vi "VideoRecording.vi"() -> ()   [LabVIEW 2015]
doc: "The LL Ring VI acquires images continuously and displays them in an image control using the low-level acquisition VIs. A ring initiates a continuous high-speed acquisition to multiple buffers and is appropriate for high-speed applications that perform processing on every image. Multiple buffers are useful when processing times vary depending on other applications and processing results .\n\nIMAQ Init initializes the device. IMAQ Configure List configures the buffer list with multiple buffers. IMAQ Create creates the image buffers. Call IMAQ Configure Buffer once for each buffer in the buffer list. IMAQ Start starts the acquisition, and IMAQ Extract Buffer ensures that the current image is not overwritten. An image control displays the image on the front panel. After exiting the loop, IMAQ Extract Buffer releases the last extracted buffer. IMAQ Close releases resources associated with the acquisition, and IMAQ Dispose frees the image buffer."
uses:
  <vilib>/vision/Avi.llb/IMAQ AVI2 Refnum.ctl
  <vilib>/vision/Avi.llb/IMAQ AVI2 Codec Path.ctl
  SubVI/Global_Video_Frame_Number.vi
panel:
  in  "Frames per file":i32=6000
  out "AVI Refnum":T1
  out "Video recording":bool=TRUE
  in  "Record? (Home bt.)":bool
  in  "codec index":i32=5
  out "Error (%)":dbl format="%#.4g"
  out "Missing Frames":i32
  out "Frame Number":u32=4950121
  out "codec":string="Y800 Uncompressed Grey Scale (NI Vision)"
  in  "AVI File Path":path=path "E:/Video/4/200fps.avi"
  out "Processed Frames/s":dbl=200.0 format="%#.1g"
  in  "Stop":bool
  out "Saved Frames":i32=21551
  out "Image":T2(plugin-control)
  in  "camera selection":string="img0"
  in  "Buffer size (frames)":u32=1000
  # "ToDo:\n - add JSON output\n - andd indicator of _s# number"
  # "1.  Initialisation"
  # "Codec should be:\n\"Y800 Uncompressed Grey Scale\""
  # "Naming convention:\n - use the name above and add _s#.avi for videos\n - specs for saved videos is specified in name.json"
  # "2.  Recording"
  # "y"
  # "Record"
  # "x"
  # "Just Observe"
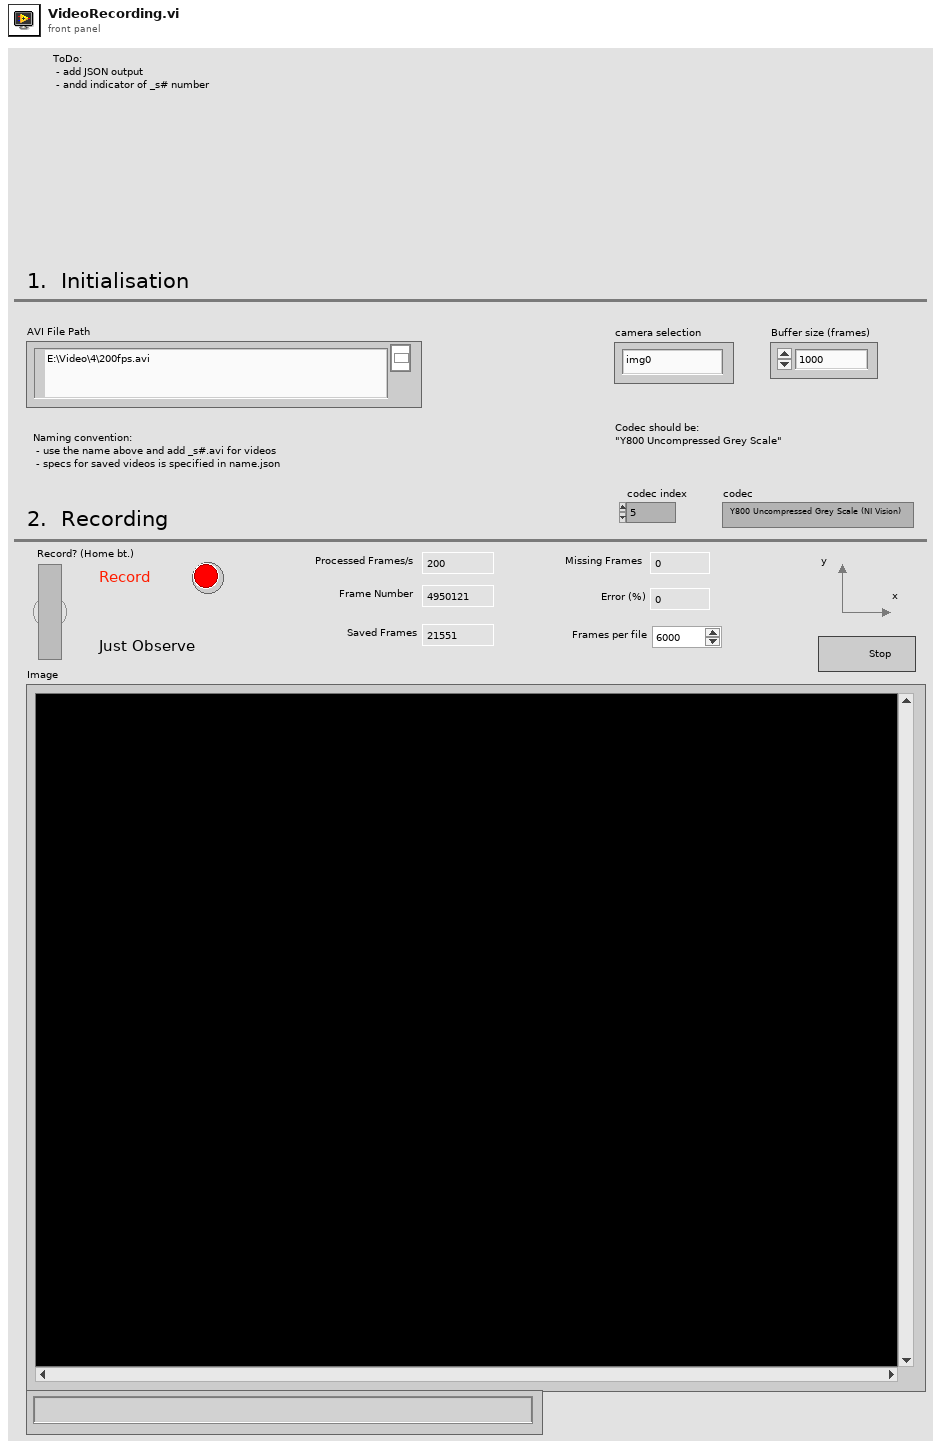
[diagram p1: front panel]
types:
  T1 = typedef "IMAQ AVI2 Refnum.ctl" = refnum<k20>
  T2 = typedef "IMAQ Image.ctl" = refnum<image>
  T3 = typedef "IMAQ AVI2 Codec Path.ctl" = u32
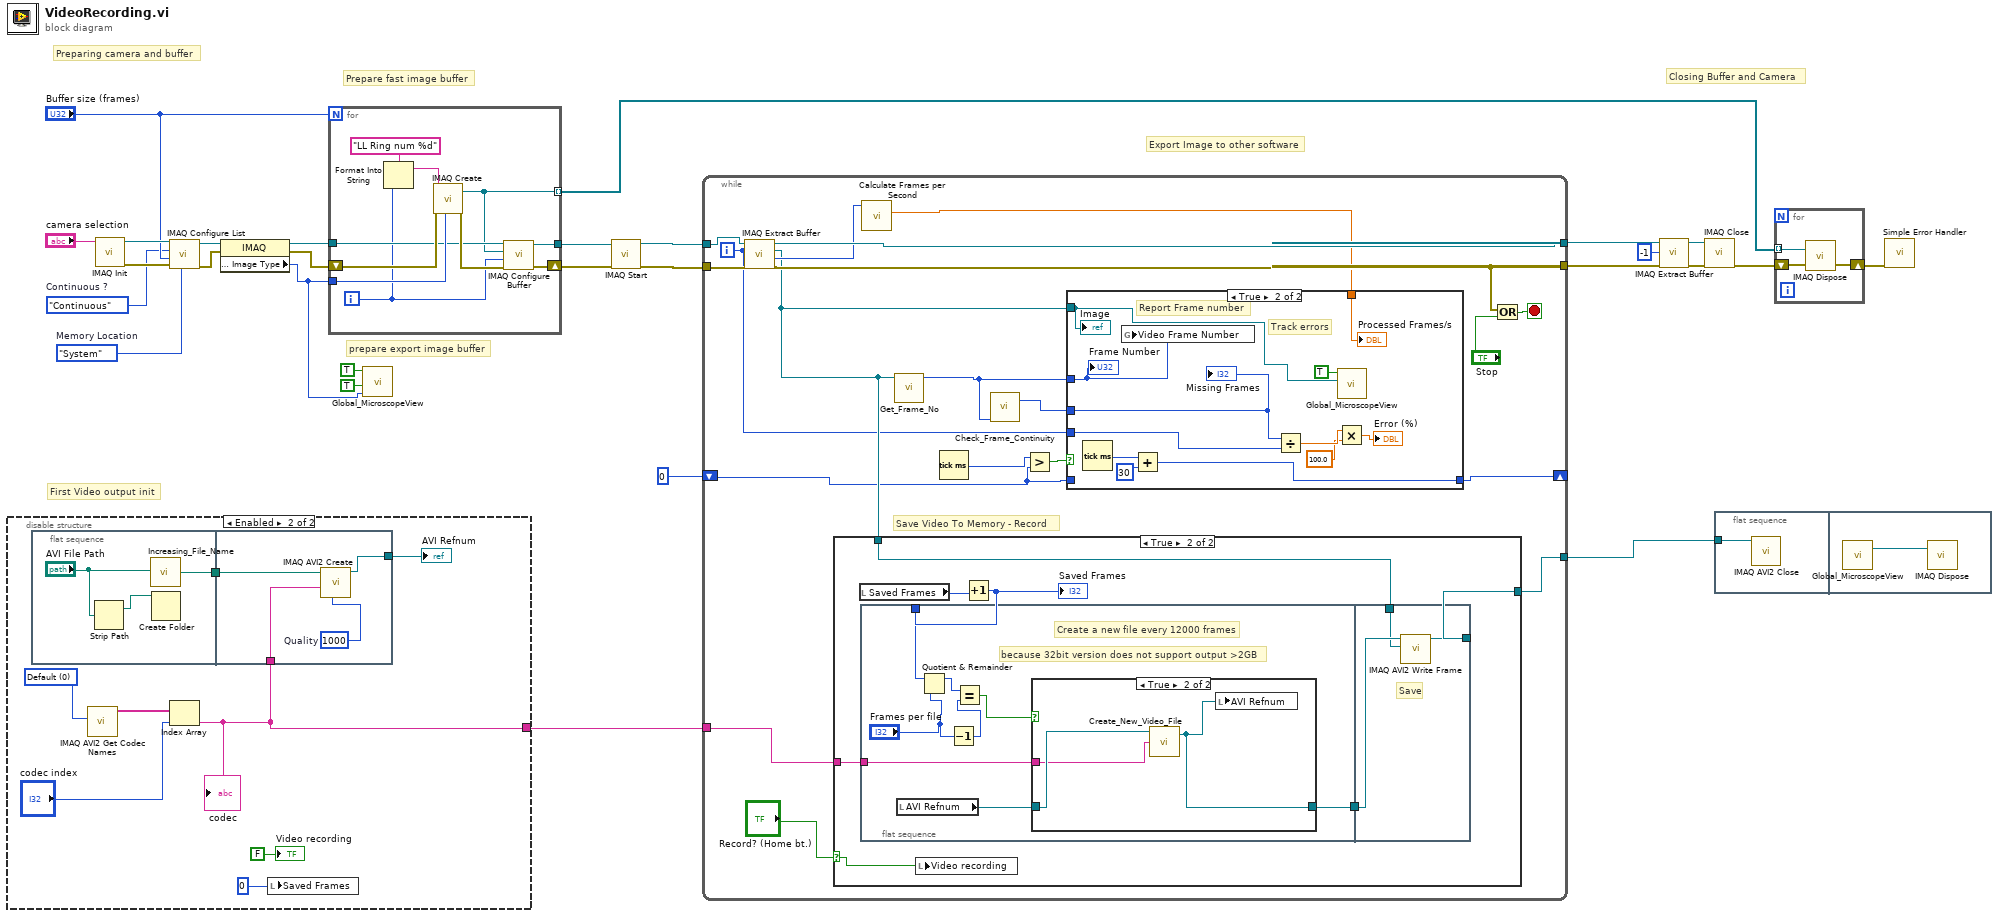
[diagram p0: block diagram]
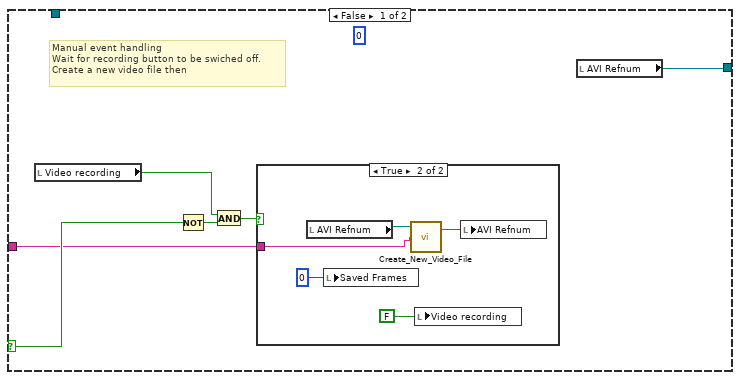
[diagram p4: hidden frame]
diagram:
  w10 = enum16{"System", "Onboard"}."System"  # Memory Location
  w9 = enum16{"One-Shot", "Continuous"}."Continuous"  # Continuous ?
  # "Export Image to other software"
  # "prepare export image buffer"
  # "Prepare fast image buffer"
  # "First Video output init"
  # "Closing Buffer and Camera"
  # "Preparing camera and buffer"
  n1 = disable-structure shown="Enabled" {
    disable-tunnel: [_ w29] -> w5
    frame Disabled {
    }
    frame Enabled {
      w36 = T3 0 items=["Default", "System", "Built in Vision"] ("Codec Source")
      n2 = flat-sequence {
        tunnel: [w39] -> w31
        tunnel: w31 -> [w41]
        tunnel: [w42] -> w30
        tunnel: w29 -> [w40]
        frame #0 {
          n3 = Strip Path(path="AVI File Path") -> (stripped path=w38:path)  [unwired: 1 out]
          n4 = call "Increasing_File_Name.vi"("Base AVI  path"="AVI File Path") -> ("Final AVI path"=w39:path)
          n5 = Create Folder(path (use dialog)=w38) -> ()  [unwired: 2 in, 3 out]
        }
        frame #1 {
          w43 = 1000  # Quality
          n6 = call "IMAQ AVI2 Create"("Quality"=w43, "Codec"=w40, "AVI Path"=w41) -> ("AVI Refnum"=w42:T1)  [unwired: 7 in, 1 out]
        }
      }
      n7 = call "IMAQ AVI2 Get Codec Names"("Codec Source"=w36) -> ("Codec Names"=w35:string[])  [unwired: 9 in, 1 out]
      n8 = Index Array(array=w35, index="codec index") -> (element=w29:string)
      "codec" <- w29
      n9 = local write "Saved Frames"(0 ("Saved Frames")) -> ()
      "AVI Refnum" <- w30
      "Video recording" <- FALSE ("Video recording")
    }
  }
  n10 = call <vilib>:"IMAQ Init.vi"("Interface Name"="camera selection") -> ("error out"=w27:errorcluster, "IMAQ Session Out"=w28:refnum<k11>)  [unwired: 1 in, 8 out]
  n11 = call <vilib>:"IMAQ Configure List.vi"("Memory Location"=w10, "error in (no error)"=w27, "Number of buffers"="Buffer size (frames)", "Continuous?"=w9, "IMAQ Session In"=w28) -> ("error out"=w23:errorcluster, "IMAQ Session Out"=w22:refnum<k11>)  [unwired: 1 in, 4 out]
  n12 = property class="IMAQ"(reference=w22, error in=w23) -> (reference out=w15:refnum<k11>, error out=w14:errorcluster, "Image Parameters : Image Type"=w2:u32)
  n13 = for {
    N: "Buffer size (frames)" -> [_]
    tunnel: [w53] -> w12
    tunnel: w2 -> [w51]
    tunnel: w15 -> [w48]
    shift-right: [w52] -> w11
    shift-left: w14 -> [w50]
    tunnel: [w44] -> w8 mode=indexing
    i -> [w45]
    n14 = Format Into String(format string="LL Ring num %d", w45) -> (resulting string=w47:string)  [unwired: 2 in, 1 out]
    n15 = call "IMAQ Create"("Image Name"=w47, "Image Type"=w51, "error in (no error)"=w50) -> ("New Image"=w44:T2, "error out"=w49:errorcluster)  [unwired: 1 in, 1 out]
    n16 = call <vilib>:"IMAQ Configure Buffer.vi"("error in (no error)"=w49, "Buffer Number"=w45, "Image In"=w44, "IMAQ Session In"=w48) -> ("error out"=w52:errorcluster, "IMAQ Session Out"=w53:refnum<k11>)  [unwired: 2 in, 4 out]
  }
  n17 = call "Global_MicroscopeView.vi"("Image Type"=w2, "Initialise"=TRUE, "Update Image"=TRUE) -> ()  [unwired: 1 in, 2 out]
  n18 = call <vilib>:"IMAQ Start.vi"("error in (no error)"=w11, "IMAQ Session In"=w12) -> ("error out"=w7:errorcluster, "IMAQ Session Out"=w18:refnum<k11>)  [unwired: 8 out]
  n19 = while {
    tunnel: [w70] -> w20
    tunnel: w18 -> [w71]
    tunnel: [w64] -> w19
    tunnel: w7 -> [w67]
    tunnel: [w63] -> w6
    tunnel: w5 -> [w62]
    shift-right: [w54] -> _
    shift-left: 0 -> [w55]
    i -> [w59]
    stop <- w72 stop-if-true
    # "Save Video To Memory - Record"
    n20 = call <vilib>:"IMAQ Extract Buffer.vi"("error in (no error)"=w67, "Buffer to extract"=w59, "IMAQ Session In"=w71) -> ("error out"=w64:errorcluster, "Buffer Number"=w68:i32, "Image Out"=w60:T2, "IMAQ Session Out"=w70:refnum<k11>)  [unwired: 5 out]
    n21 = case shown="True" "Record? (Home bt.)" {
      selector: "Record? (Home bt.)" -> [w88 w99]
      tunnel: [w91 w102] -> w63
      tunnel: w60 -> [_ w100]
      tunnel: w62 -> [w86 w98]
      frame False {
        (unwired) 0
        # "Manual event handling\nWait for recording button to be swiched off.\nCreate a new video file then"
        n22 = local read "Video recording"() -> (w87:bool)
        n23 = Not(x=w88) -> (.not. x?=w89:bool)
        n24 = And(x=w87, y=w89) -> (x .and. y?=w90:bool)
        n25 = case shown="True" w90 {
          tunnel: w86 -> [_ w92]
          frame False {
          }
          frame True {
            n26 = local read "AVI Refnum"() -> (w95:T1)
            n27 = local write "Saved Frames"(0 ("Saved Frames")) -> ()
            n28 = call "Create_New_Video_File.vi"("Codec"=w92, "AVI Refnum IN"=w95) -> ("AVI Refnum OUT"=w96:T1)  [unwired: 1 in, 1 out]
            n29 = local write "Video recording"(FALSE ("Video recording")) -> ()
            n30 = local write "AVI Refnum"(w96) -> ()
          }
        }
        n31 = local read "AVI Refnum"() -> (w91:T1)
      }
      frame True {
        n32 = local read "Saved Frames"() -> (w103:i32)
        n33 = flat-sequence {
          tunnel: w97 -> [w109]
          tunnel: [w106] -> w101
          tunnel: w98 -> [w105]
          tunnel: [w118] -> w102
          tunnel: w101 -> [w117]
          tunnel: w100 -> [w116]
          frame #0 {
            # "because 32bit version does not support output >2GB"
            # "Create a new file every 12000 frames"
            n34 = local read "AVI Refnum"() -> (w107:T1)
            n35 = Quotient & Remainder(x=w109, y="Frames per file") -> (x-y*floor(x/y)=w111:i32)  [unwired: 1 out]
            n36 = Decrement(x="Frames per file") -> (x-1=w110:i32)
            n37 = Equal?(x=w111, y=w110) -> (x = y?=w108:bool)
            n38 = case shown="True" w108 {
              tunnel: w107 -> [w112 w115]
              tunnel: [w112 w114] -> w106
              tunnel: w105 -> [_ w113]
              frame False {
              }
              frame True {
                n39 = call "Create_New_Video_File.vi"("Codec"=w113, "AVI Refnum IN"=w115) -> ("AVI Refnum OUT"=w114:T1)  [unwired: 1 in, 1 out]
                n40 = local write "AVI Refnum"(w114) -> ()
              }
            }
          }
          frame #1 {
            # "Save"
            n41 = call "IMAQ AVI2 Write Frame"("Image"=w116, "AVI Refnum"=w117) -> ("AVI Refnum (duplicate)"=w118:T1)  [unwired: 7 in, 2 out]
          }
        }
        n42 = local write "Video recording"(w99) -> ()
        n43 = Increment(x=w103) -> (x+1=w97:i32)
        "Saved Frames" <- w97
      }
    }
    n44 = call <vilib>:"Calculate Frames per Second.vi"("Buffer Number"=w68) -> ("Processed Frames/s"=w58:dbl)  [unwired: 8 in, 2 out]
    n45 = call "Get_Frame_No.vi"("Image In"=w60) -> ("Frame Number"=w61:u32)  [unwired: 10 in]
    n46 = Tick Count (ms)() -> (millisecond timer value=w56:u32)
    n47 = call "Check_Frame_Continuity.vi"("N"=w61) -> ("No of missed frames"=w66:i32)  [unwired: 1 in, 1 out]
    n48 = Greater?(x=w56, y=w55) -> (0:w57:bool)
    n49 = case shown="True" w57 {
      tunnel: w66 -> [_ w82]
      tunnel: w59 -> [_ w81]
      tunnel: w61 -> [_ w80]
      tunnel: w60 -> [_ w75]
      tunnel: w58 -> [_ w79]
      tunnel: w55 -> [w73 _]
      tunnel: [w73 w77] -> w54
      frame False {
      }
      frame True {
        # "Track errors"
        # "Report Frame number"
        n50 = Tick Count (ms)() -> (millisecond timer value=w78:u32)
        n51 = global write "Global_Video_Frame_Number.vi" "Video Frame Number"(w80) -> ()
        n52 = Add(x=w78, y=u32 30) -> (x+y=w77:u32)
        n53 = Divide(x=w82, y=w81) -> (x/y=w84:dbl)
        n54 = call "Global_MicroscopeView.vi"("New Image"=w75, "Update Image"=TRUE) -> ()  [unwired: 2 in, 2 out]
        n55 = Multiply(x=w84, y=100.0) -> (x*y=→"Error (%)":dbl)
        "Frame Number" <- w80
        "Missing Frames" <- w82
        "Image" <- w75
        "Processed Frames/s" <- w79
      }
    }
    n56 = Or(x=w64, y="Stop") -> (x .or. y?=w72:bool)
  }
  n57 = call <vilib>:"IMAQ Extract Buffer.vi"("error in (no error)"=w19, "Buffer to extract"=-1, "IMAQ Session In"=w20) -> ("error out"=w17:errorcluster, "IMAQ Session Out"=w16:refnum<k11>)  [unwired: 7 out]
  n58 = call <vilib>:"IMAQ Close.vi"("error in (no error)"=w17, "IMAQ Session In"=w16) -> ("error out"=w24:errorcluster)  [unwired: 9 out]
  n59 = flat-sequence {
    tunnel: w6 -> [w119]
    frame #0 {
      n60 = call "IMAQ AVI2 Close"("AVI Refnum"=w119) -> ()  [unwired: 10 in, 1 out]
    }
    frame #1 {
      n61 = call "Global_MicroscopeView.vi"() -> ("MicroscopeView"=w120:T2)  [unwired: 4 in, 1 out]
      n62 = call "IMAQ Dispose"("Image"=w120) -> ()  [unwired: 2 in, 4 out]
    }
  }
  n63 = for {
    tunnel: w8 -> [w123] mode=indexing
    shift-right: [w121] -> w25
    shift-left: w24 -> [w122]
    n64 = call "IMAQ Dispose"("Image"=w123, "error in (no error)"=w122) -> ("error out"=w121:errorcluster)  [unwired: 1 in, 3 out]
  }
  n65 = call <vilib>:"Simple Error Handler.vi"("error in (no error)"=w25) -> ()  [unwired: 1 in, 8 out]
